vi "Init.vi"(7 "I2C":T2=-1, 8 "error in (no error)":errorcluster, 10 "Session":refnum<class "Session.lvclass">, 11 "Address":T1 format="%02x") -> (0 "error out":errorcluster, 3 "I2C Peripheral":refnum<class "I2C Connection.lvclass">)   [LabVIEW 2020, in "CTI.lvlib" / "I2C Connection.lvclass"]
uses:
  I2C Connection.lvclass
  I2C Number.ctl
  I2C Address.ctl
  Session/Session.lvclass
  I2C Connection.lvclass/I2C Connection.ctl
  CTI.lvlib
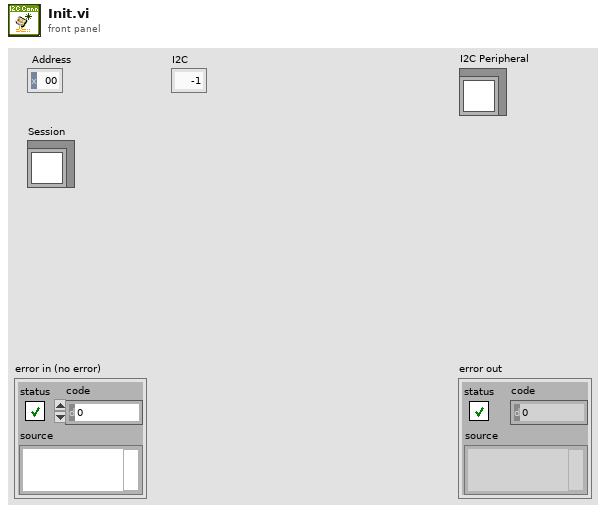
[diagram p1: front panel]
types:
  T1 = typedef "CTI.lvlib/I2C Address.ctl" = u8
  T2 = typedef "CTI.lvlib/I2C Number.ctl" = i8
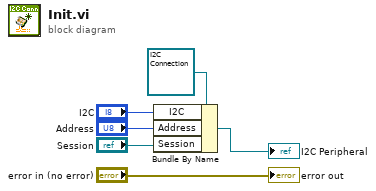
[diagram p0: block diagram]
diagram:
  n1 = Bundle By Name(cluster=refnum<class "I2C Connection.lvclass"> refnum ("I2C Device in"), "I2C"="I2C", "Address"="Address", "Session"="Session") -> (→"I2C Peripheral":refnum<class "I2C Connection.lvclass">)
  "error out" <- "error in (no error)"
